vi "Generate-Sound-PC-Out-WN.vi"() -> ()   [LabVIEW 2022 SP3]
doc: "This VI illustrates how to generate and play sine, square, sawtooth and triangle waveforms. You can change the frequency and type of the waveform generated as it plays continuously."
uses:
  <vilib>/sound2/lvsound2.llb/Sampling Mode.ctl
  <vilib>/sound2/lvsound2.llb/Sound Data Format.ctl
  <vilib>/Analysis/4window.llb/windowTd.ctl
  <vilib>/sound2/lvsound2.llb/Sound Output Set Volume (Single).vi
  <vilib>/measure/NI_MAPro.lvlib
  <vilib>/Analysis/NI_AALPro.lvlib
  <vilib>/measure/NI_MABase.lvlib
  <vilib>/measure/matone.llb/Extract Single Tone Information 1 Chan.vi
  <vilib>/sound2/lvsound2.llb/Sound Output Write (DBL Single).vi
  <vilib>/measure/maspectr.llb/FFT Spectrum (Mag-Phase) for 1 Chan.vi
panel:
  in  "Lower Cut-Off":dbl=300.0
  out "detected amplitudes":dbl[](array[numeric]) format="%.2p"
  out "detected frequencies":dbl[](array[numeric]) format="%.2p"
  out "FFT":cluster{"f0":dbl, "df":dbl, "magnitude":dbl[]}(graph)
  in  "Volume":dbl(slide)=50.0 scale=0.0..100.0
  out "Generated Sound":waveform(dbl)(graph)
  in  "Standard Deviation":dbl=1.0
  in  "Stop":bool
  in  "Device ID":u32
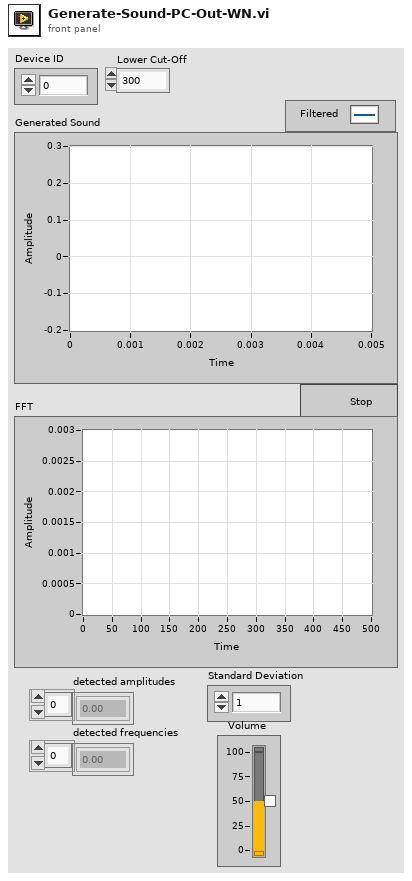
[diagram p1: front panel]
types:
  T1 = typedef "Sound Data Format.ctl" = cluster{"sample rate (S/s)":dbl, "number of channels":i32, "bits per sample":i32}
  T2 = typedef "Sampling Mode.ctl" = i32
  T3 = typedef "Sound Output Task ID.ctl" = u32
  T4 = cluster{"averaging mode":enum16{"No averaging", "Vector averaging", "RMS averaging", "Peak hold"}, "weighting mode":enum16{"Linear", "Exponential"}, "number of averages":u32}
  T5 = cluster{"dB On (F)":bool, "unwrap phase (F)":bool, "convert to degree (F)":bool}
  T6 = typedef "NI_AALPro.lvlib/windowTd.ctl" = u32
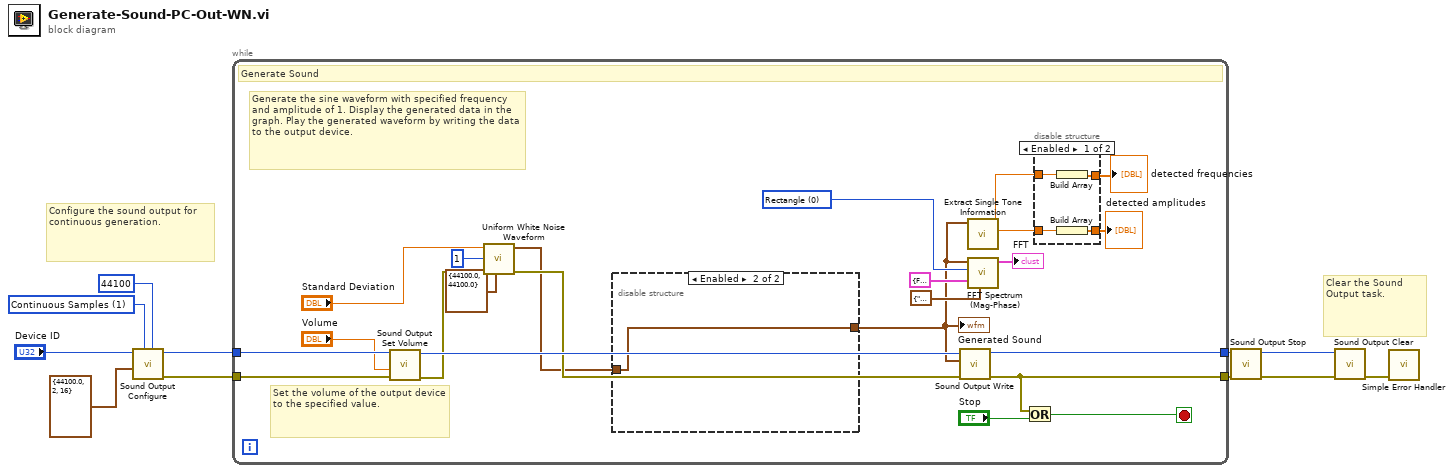
[diagram p0: block diagram]
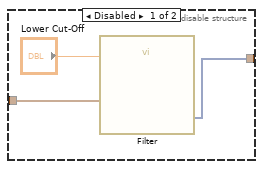
[diagram p3: hidden frame]
diagram:
  w7 = T2 1 items=["Finite Samples", "Continuous Samples"] ("sample mode")
  # "Configure the sound output for continuous generation."
  # "Clear the Sound Output task."
  n1 = call <vilib>:"Sound Output Configure.vi"("number of samples/ch"=44100 ("Number of Samples/ch"), "sample mode"=w7, "sound format"=T1 {"sample rate (S/s)"=44100.0, "number of channels"=2, "bits per sample"=16} ("Sound Format"), "device ID"="Device ID") -> ("error out"=w11:errorcluster, "task ID"=w10:T3)  [unwired: 6 in]
  n2 = while {
    tunnel: w10 -> [w31]
    tunnel: [w34] -> w9
    tunnel: w11 -> [w32]
    tunnel: [w30] -> w2
    stop <- w33 stop-if-true
    w21 = T6 0 items=["Rectangle"=0, "Hanning"=1, "Hamming"=2, "Blackman-Harris"=3, "Exact Blackman"=4, "Blackman"=5, "Flat Top"=6, "4 Term B-Harris "=7, "7 Term B-Harris"=8, "Low Sidelobe"=9, "Blackman Nuttall"=11, "Triangle"=30, "Bartlett-Hanning"=31, "Bohman"=32, "Parzen"=33, "Welch"=34, "Kaiser"=60, "Dolph-Chebyshev"=61, "Gaussian"=62] ("window")
    # "Set the volume of the output device to the specified value."
    # "Generate the sine waveform with specified frequency and amplitude of 1. Display the generated data in the graph. Play the generated waveform by writing the data to the output device."
    # "Generate Sound"
    n3 = call-poly <vilib>:"Sound Output Set Volume.vi"("error in (no error)"=w32, "volume"="Volume", "task ID"=w31) -> ("error out"=w26:errorcluster, "task ID out"=w28:T3)  [unwired: 7 in]
    n4 = call <vilib>:"Uniform White Noise Waveform.vi"("sampling info"=cluster{"Fs":dbl, "#s":dbl} {"Fs"=44100.0, "#s"=44100.0}, "error in (no error)"=w26, "seed"=1, "amplitude"="Standard Deviation") -> ("error out"=w25:errorcluster, "signal out"=w17:waveform(dbl))  [unwired: 6 in]
    n5 = disable-structure shown="Enabled" {
      disable-tunnel: w17 -> [w43 w44]
      disable-tunnel: [w42 w44] -> w16
      frame Disabled {
        n6 = call "Filter"("Lower Cut-Off"="Lower Cut-Off", "Signal"=w43) -> ("Filtered Signal"=w42:dynamicdata)  [unwired: 8 in, 1 out]
      }
      frame Enabled {
      }
    }
    "Generated Sound" <- w16
    n7 = call-poly <vilib>:"Sound Output Write.vi"("error in (no error)"=w25, "data"=w16, "task ID"=w28) -> ("error out"=w30:errorcluster, "task ID out"=w34:T3)  [unwired: 7 in]
    n8 = call-poly <vilib>:"Extract Single Tone Information.vi"("time signal in"=w16) -> ("detected amplitude"=w14:dbl, "detected frequency"=w15:dbl)  [unwired: 5 in, 4 out]
    n9 = call-poly <vilib>:"FFT Spectrum (Mag-Phase).vi"("averaging parameters"=T4 {"averaging mode"=enum."Vector averaging", "weighting mode"=enum."Linear", "number of averages"=10}, "view"=T5 {"dB On (F)"=FALSE, "unwrap phase (F)"=FALSE, "convert to degree (F)"=FALSE}, "window"=w21, "time signal"=w16) -> ("magnitude"=→"FFT":cluster{"f0":dbl, "df":dbl, "magnitude":dbl[]})  [unwired: 3 in, 4 out]
    n10 = Or(x=w30, y="Stop") -> (x .or. y?=w33:bool)
    n11 = disable-structure shown="Enabled" {
      disable-tunnel: w15 -> [w38 w40]
      disable-tunnel: w14 -> [w37 w39]
      disable-tunnel: [w36 w40] -> w13
      disable-tunnel: [w35 w39] -> w12
      frame Enabled {
        n12 = Build Array(w38) -> (w36:dbl[])
        n13 = Build Array(w37) -> (w35:dbl[])
      }
      frame Disabled {
      }
    }
    "detected frequencies" <- w13
    "detected amplitudes" <- w12
  }
  n14 = call <vilib>:"Sound Output Stop.vi"("error in (no error)"=w2, "task ID"=w9) -> ("error out"=w1:errorcluster, "task ID out"=w3:T3)  [unwired: 8 in]
  n15 = call <vilib>:"Sound Output Clear.vi"("error in (no error)"=w1, "task ID"=w3) -> ("error out"=w5:errorcluster)  [unwired: 9 in]
  n16 = call <vilib>:"Simple Error Handler.vi"("error in (no error)"=w5) -> ()  [unwired: 4 in, 5 out]
